vi "FindSNK3 (SubVI).vi"(11 "String in":refnum<vi>) -> (0 "error out":errorcluster, 3 "Cancel":bool)   [LabVIEW 2017]
uses:
  Global_SNK3_HF.vi
  E:/_git/LV_Unicorn/LV_Unicorn.lvlib
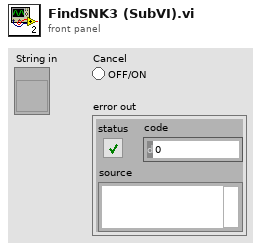
[diagram p1: front panel]
types:
  T1 = typedef "LV_Unicorn.lvlib/AnswerUDP.ctl" = cluster{"IP":string, "Port":u16, "DataVersion":u16, "ModbusAddress":i32, "type_version":string, "Description":string, "Serial":string, "ServerPort":u16}
  T2 = typedef "LV_Unicorn.lvlib/unicorn_Param.ctl" = cluster{"conParam":T3, "Param":T4}
  T3 = typedef "LV_Unicorn.lvlib/unicorn_conn.ctl" = cluster{"ReadIntParam":bool, "ReadDescrParam":bool, "ReadFloatParam":bool, "debug":bool, "ReadJSON":bool, "IP_address":string, "N_attempts":i32, "type_con":enum16{"Serial", "TCP"}, "MB_address":i32, "VISA":refnum<visa-resource-name>, "connection ID":refnum<k5>, "nameDevices":string, "timeout":i32, "port":u16, "type_version":string, "baud_rate":u32, "VersionControl":bool, "TCP_conn":bool, "WindowSize":i32}
  T4 = typedef "LV_Unicorn.lvlib/unicorn_JSON.ctl" = cluster{"NumParam":cluster{"NTelem":i32, "NInt":i32, "NFloat":i32, "NTable":i32}, "ParamInt":T5, "Telemetry":T6, "Table":T7, "ParamFloat":T8}
  T5 = typedef "LV_Unicorn.lvlib/unicorn_ParamInt.ctl" = cluster{"ID":string, "Num":i32, "Name":string, "Type":string, "Enum":string, "Desc":string, "Unit":string, "Access":string, "FormatStr":string, "Min":i32, "Max":i32}[]
  T6 = typedef "LV_Unicorn.lvlib/unicorn_Telemetry.ctl" = cluster{"ID":string, "Num":i32, "Name":string, "Desc":string, "Unit":string, "FormatStr":string, "Min":i32, "Max":i32}[]
  T7 = typedef "LV_Unicorn.lvlib/unicorn_Table.ctl" = cluster{"Num":i32, "Access":string, "ColumnCount":i32, "NeedParamPrepare":bool, "Columns":cluster{"Column":i32, "Desc":string, "Name":string}[], "DataType":string, "FormatStr":string, "ID":string, "Name":string, "RowCount":i32, "Rows":cluster{"Desc":string, "ID":string, "Max":i32, "Min":i32, "Name":string, "Row":i32, "Unit":string}[], "Type":string}[]
  T8 = typedef "LV_Unicorn.lvlib/unicorn_ParamFloat.ctl" = cluster{"ID":string, "Num":i32, "Name":string, "Type":string, "Enum":string, "Desc":string, "Unit":string, "Access":string, "FormatStr":string, "Min":sgl, "Max":sgl}[]
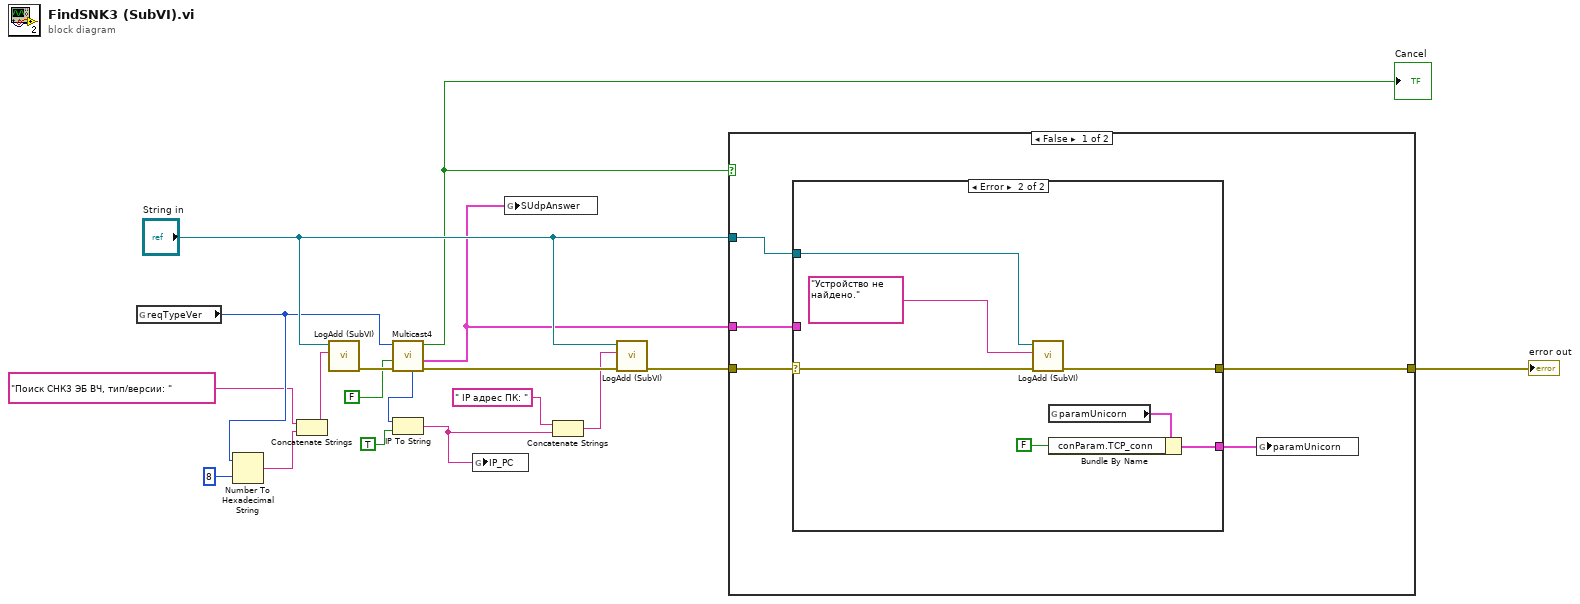
[diagram p0: block diagram]
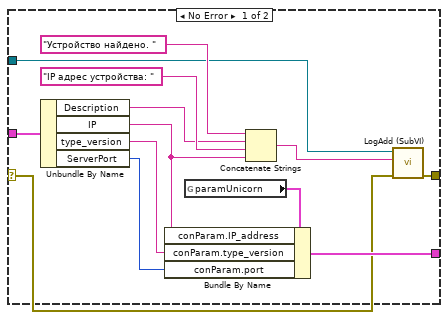
[diagram p2: hidden frame]
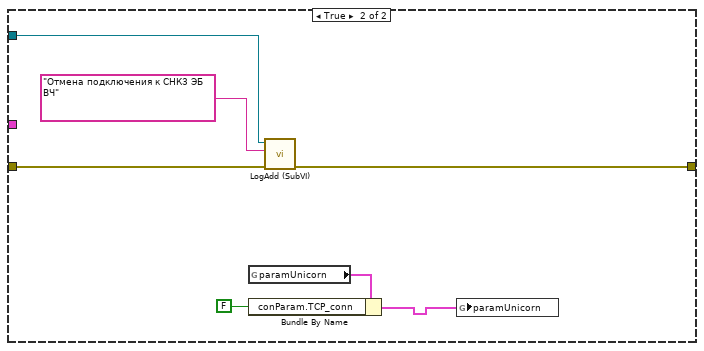
[diagram p3: hidden frame]
diagram:
  n1 = global read "Global_SNK3_HF.vi" "reqTypeVer"() -> (w4:i32)
  n2 = Number To Hexadecimal String(1:i16 8 ("width (-)"), 2:w4) -> (0:w5:string)
  n3 = Concatenate Strings("Поиск СНК3 ЭБ ВЧ, тип/версии: " ("string"), w5) -> (w2:string)
  n4 = call "LogAdd (SubVI).vi"("string"=w2, "Log"="String in") -> ("error out"=w14:errorcluster)  [unwired: 9 in]
  n5 = call "Multicast4.vi"("error in"=w14, "VersionControl"=FALSE, "type_version"=w4) -> ("error out"=w15:errorcluster, "selDevice"=w13:T1, "Cancel"=w1:bool, "selIPhex"=w11:u32)  [unwired: 3 in, 2 out]
  "Cancel" <- w1
  n6 = IP To String(1:TRUE ("dot notation? (F)"), 2:w11) -> (0:w10:string)
  n7 = global write "Global_SNK3_HF.vi" "IP_PC"(w10) -> ()
  n8 = global write "Global_SNK3_HF.vi" "SUdpAnswer"(w13) -> ()
  n9 = Concatenate Strings(" IP адрес ПК: " ("string"), w10) -> (w7:string)
  n10 = call "LogAdd (SubVI).vi"("error in"=w15, "string"=w7, "Log"="String in") -> ("error out"=w16:errorcluster)  [unwired: 8 in]
  n11 = case shown="False" w1 {
    tunnel: "String in" -> [w23 w45]
    tunnel: [w22 w46] -> w17
    tunnel: w16 -> [w21 w47]
    tunnel: w13 -> [w19 _]
    frame False {
      n12 = case shown="Error" w21 {
        selector: w21 -> [w26 w39]
        tunnel: w19 -> [w32 _]
        tunnel: [w27 w41] -> w20
        tunnel: [w25 w38] -> w22
        tunnel: w23 -> [w24 w37]
        frame No Error {
          n13 = Unbundle By Name(w32) -> ("Description"=w31:string, "IP"=w30:string, "type_version"=w29:string, "ServerPort"=w28:u16)
          n14 = global read "Global_SNK3_HF.vi" "paramUnicorn"() -> (w33:T2)
          n15 = Bundle By Name(cluster=w33, "conParam.IP_address"=w30, "conParam.type_version"=w29, "conParam.port"=w28) -> (w27:T2)
          n16 = Concatenate Strings("Устройство найдено. " ("string"), w31, "IP адрес устройства: " ("string"), w30) -> (w35:string)
          n17 = call "LogAdd (SubVI).vi"("error in"=w26, "string"=w35, "Log"=w24) -> ("error out"=w25:errorcluster)  [unwired: 8 in]
        }
        frame Error {
          n18 = call "LogAdd (SubVI).vi"("error in"=w39, "string"="Устройство не найдено.", "Log"=w37) -> ("error out"=w38:errorcluster)  [unwired: 8 in]
          n19 = global read "Global_SNK3_HF.vi" "paramUnicorn"() -> (w42:T2)
          n20 = Bundle By Name(cluster=w42, "conParam.TCP_conn"=FALSE) -> (w41:T2)
        }
      }
      n21 = global write "Global_SNK3_HF.vi" "paramUnicorn"(w20) -> ()
    }
    frame True {
      n22 = global read "Global_SNK3_HF.vi" "paramUnicorn"() -> (w49:T2)
      n23 = Bundle By Name(cluster=w49, "conParam.TCP_conn"=FALSE) -> (w50:T2)
      n24 = call "LogAdd (SubVI).vi"("error in"=w47, "string"="Отмена подключения к СНК3 ЭБ ВЧ", "Log"=w45) -> ("error out"=w46:errorcluster)  [unwired: 8 in]
      n25 = global write "Global_SNK3_HF.vi" "paramUnicorn"(w50) -> ()
    }
  }
  "error out" <- w17
